vi "Triggered Data Acquisition.vi"(8 "error in":errorcluster, 11 "4300 in":refnum<class "4300.lvclass">) -> (0 "error out":errorcluster, 2 "Timeout?":bool, 3 "4300 out":refnum<class "4300.lvclass">)   [LabVIEW 2019, in "4300.lvlib" / "4300.lvclass"]
uses:
  Library/4300.lvclass
  C:/Users/Public/Documents/Development/builds/Instruments/AnalogInput.lvlibp/Library/AnalogInput.lvclass
  C:/Users/Public/Documents/Development/builds/Instruments/Instruments.lvlibp/Library/Instruments.lvclass
  Library/4300.lvclass/4300.ctl
  <vilib>/DAQmx/read.llb/DAQmx Read (Analog 1D Wfm NChan NSamp).vi
  builds/Instruments/AnalogInput.lvlibp/Accessors/Triggering/Read Trigger Settings.vi
  <vilib>/DAQmx/miscellaneous.llb/DAQmx Fill In Error Info.vi
  builds/Instruments/AnalogInput.lvlibp/Accessors/Write Timeout Event.vi
  builds/Instruments/Instruments.lvlibp/Accessors/Write Snapshot.vi
  builds/Instruments/AnalogInput.lvlibp/Accessors/Read Timeout Event.vi
  builds/Instruments/AnalogInput.lvlibp/Accessors/Triggering/Write Snapshot_Timeout.vi
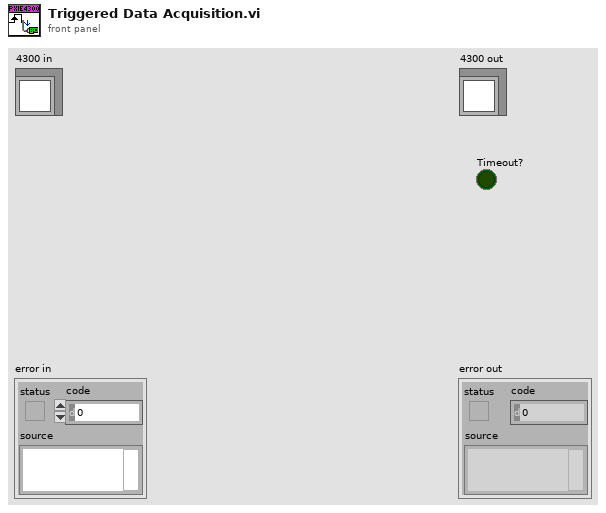
[diagram p1: front panel]
types:
  T1 = typedef "AnalogInput.lvlibp/AnalogInput.lvclass/User Trigger Settings.ctl" = cluster{"Timeout":dbl, "Level":dbl, "Slope":T2, "samples per channel":i32, "Sample Rate (10k)":dbl, "pretrigger samples":u32}
  T2 = typedef "AnalogInput.lvlibp/AnalogInput.lvclass/Trigger_Slope.ctl" = enum16{"Rising", "Falling"}
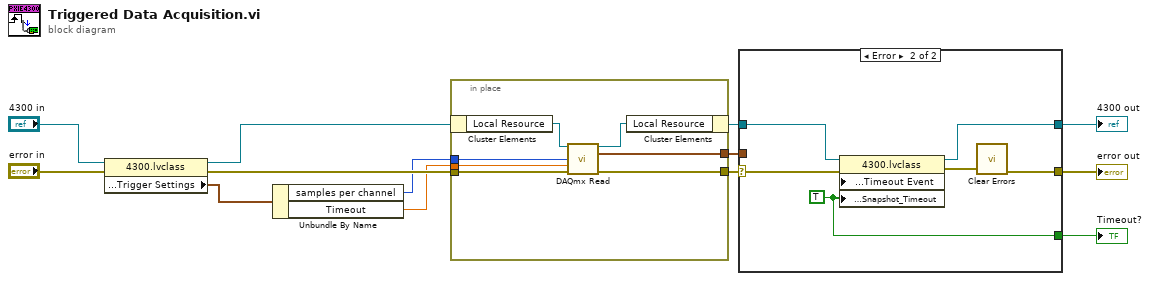
[diagram p0: block diagram]
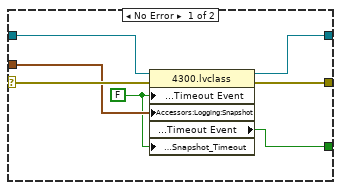
[diagram p2: hidden frame]
diagram:
  n1 = property class="4300.lvclass"(reference="4300 in", error in="error in") -> (reference out=w2:refnum<class "4300.lvclass">, error out=w13:errorcluster, "Accessors:Triggering:Trigger Settings"=w10:T1)
  n2 = Unbundle By Name(w10) -> ("samples per channel"=w4:i32, "Timeout"=w9:dbl)
  n3 = in-place {
    in-place-border: w13 -> [w20]
    in-place-border: [w19] -> w12
    in-place-border: [w18] -> w11
    in-place-border: w9 -> [w17]
    in-place-border: w4 -> [w16]
    n4 = in-place-cluster #1(w2) -> ("Local Resource"=w15:refnum<k21>)
    n5 = call-poly <vilib>:"DAQmx Read.vi"("task/channels in"=w15, "number of samples per channel"=w16, "timeout"=w17, "error in"=w20) -> ("task out"=w14:refnum<k21>, "data"=w18:waveform(dbl)[], "error out"=w19:errorcluster)  [unwired: 9 in]
    n6 = in-place-cluster #1("Local Resource"=w14) -> (w1:refnum<class "4300.lvclass">)
  }
  n7 = case shown="Error" w12 {
    selector: w12 -> [w26 w30]
    tunnel: w1 -> [w27 w32]
    tunnel: w11 -> [w23 _]
    tunnel: [w25 w31] -> w5
    tunnel: [w24 w33] -> w3
    tunnel: [w22 w28] -> w7
    frame No Error {
      w21 = FALSE ("Timeout Event")
      n8 = property class="4300.lvclass"(reference=w27, error in=w26, "Accessors:Triggering:Timeout Event"=w21, "Accessors:Logging:Snapshot"=w23, "Accessors:Triggering:Snapshot_Timeout"=w21) -> (reference out=w25:refnum<class "4300.lvclass">, error out=w24:errorcluster, "Accessors:Triggering:Timeout Event"=w22:bool)
    }
    frame Error {
      w28 = TRUE ("Timeout Event")
      n9 = property class="4300.lvclass"(reference=w32, error in=w30, "Accessors:Triggering:Timeout Event"=w28, "Accessors:Triggering:Snapshot_Timeout"=w28) -> (reference out=w31:refnum<class "4300.lvclass">, error out=w29:errorcluster)
      n10 = call <vilib>:"Clear Errors.vi"("error in (no error)"=w29) -> ("error out"=w33:errorcluster)  [unwired: 5 in, 1 out]
    }
  }
  "error out" <- w3
  "4300 out" <- w5
  "Timeout?" <- w7
